vi "全局F参数.vi"() -> ()   [LabVIEW 2018]
panel:
  in  "选项卡控件":enum32{"1#", "2#", "3#"}(tab)
  in  "1#轮盘关开Pr":T1={"选择"=enum."Fx", "系数x"=1.0, "系数+"=1.0, "上限"=4.3, "下限"=3.7, "Ymax"=50.0, "Ymin"=-50.0, "点数"=1000.0, "锁系数x"=1.0, "锁上限"=0.4, "锁下限"=0.6, "锁系数+"=1.0, "起点"=0.20000000298023224, "终点"=0.6499999761581421, "锁起点"=0.05000000074505806, "锁终点"=0.20000000298023224, "上参考"=4.3, "下参考"=3.7, "基准"=3.7} {"系数+" format="%.3f"; "基准" format="%.2f"; "下参考" format="%.2f"; "上参考" format="%.2f"; "锁终点" format="%.2f"; "锁起点" format="%.2f"; "终点" format="%.2f"; "起点" format="%.2f"; "锁系数+" format="%.3f"; "锁下限" format="%.2f"; "锁上限" format="%.2f"; "锁系数x" format="%.3f"; "下限" format="%.2f"; "上限" format="%.2f"; "系数x" format="%.3f"}
  in  "1#轮盘开关Pr":T1={"选择"=enum."Fx", "系数x"=1.0, "系数+"=1.0, "上限"=4.3, "下限"=3.7, "Ymax"=50.0, "Ymin"=-50.0, "点数"=1000.0, "锁系数x"=1.0, "锁上限"=0.4, "锁下限"=0.6, "锁系数+"=1.0, "起点"=0.20000000298023224, "终点"=0.6499999761581421, "锁起点"=0.05000000074505806, "锁终点"=0.20000000298023224, "上参考"=4.3, "下参考"=3.7, "基准"=3.7} {"系数+" format="%.3f"; "基准" format="%.2f"; "下参考" format="%.2f"; "上参考" format="%.2f"; "锁终点" format="%.2f"; "锁起点" format="%.2f"; "终点" format="%.2f"; "起点" format="%.2f"; "锁系数+" format="%.3f"; "锁下限" format="%.2f"; "锁上限" format="%.2f"; "锁系数x" format="%.3f"; "下限" format="%.2f"; "上限" format="%.2f"; "系数x" format="%.3f"}
  in  "1#拨钮右左Pr":T1={"选择"=enum."Fx", "系数x"=1.0, "系数+"=1.0, "上限"=2.55, "下限"=2.05, "Ymax"=5.0, "Ymin"=-5.0, "点数"=1000.0, "锁系数x"=1.0, "锁上限"=0.4, "锁下限"=0.6, "锁系数+"=1.0, "起点"=0.0, "终点"=0.0, "锁起点"=0.05000000074505806, "锁终点"=0.20000000298023224, "上参考"=4.3, "下参考"=3.7, "基准"=3.7} {"系数+" format="%.3f"; "锁终点" format="%.2f"; "锁起点" format="%.2f"; "锁系数+" format="%.3f"; "锁下限" format="%.2f"; "锁上限" format="%.2f"; "锁系数x" format="%.3f"; "基准" format="%.2f"; "下参考" format="%.2f"; "上参考" format="%.2f"; "终点" format="%.2f"; "起点" format="%.2f"; "下限" format="%.2f"; "上限" format="%.2f"; "系数x" format="%.3f"}
  in  "1#拨钮左右Pr":T1={"选择"=enum."Fx", "系数x"=1.0, "系数+"=1.0, "上限"=2.55, "下限"=2.05, "Ymax"=5.0, "Ymin"=-5.0, "点数"=1000.0, "锁系数x"=1.0, "锁上限"=0.4, "锁下限"=0.6, "锁系数+"=1.0, "起点"=0.0, "终点"=0.0, "锁起点"=0.05000000074505806, "锁终点"=0.20000000298023224, "上参考"=4.3, "下参考"=3.7, "基准"=3.7} {"系数+" format="%.3f"; "锁终点" format="%.2f"; "锁起点" format="%.2f"; "锁系数+" format="%.3f"; "锁下限" format="%.2f"; "锁上限" format="%.2f"; "锁系数x" format="%.3f"; "基准" format="%.2f"; "下参考" format="%.2f"; "上参考" format="%.2f"; "终点" format="%.2f"; "起点" format="%.2f"; "下限" format="%.2f"; "上限" format="%.2f"; "系数x" format="%.3f"}
  in  "1#拨钮下上Pr":T1={"选择"=enum."Fx", "系数x"=1.0, "系数+"=1.0, "上限"=2.55, "下限"=2.05, "Ymax"=5.0, "Ymin"=-5.0, "点数"=1000.0, "锁系数x"=1.0, "锁上限"=0.4, "锁下限"=0.6, "锁系数+"=1.0, "起点"=0.0, "终点"=0.0, "锁起点"=0.05000000074505806, "锁终点"=0.20000000298023224, "上参考"=4.3, "下参考"=3.7, "基准"=3.7} {"系数+" format="%.3f"; "锁终点" format="%.2f"; "锁起点" format="%.2f"; "锁系数+" format="%.3f"; "锁下限" format="%.2f"; "锁上限" format="%.2f"; "锁系数x" format="%.3f"; "基准" format="%.2f"; "下参考" format="%.2f"; "上参考" format="%.2f"; "终点" format="%.2f"; "起点" format="%.2f"; "下限" format="%.2f"; "上限" format="%.2f"; "系数x" format="%.3f"}
  in  "1#拨钮上下Pr":T1={"选择"=enum."Fx", "系数x"=1.0, "系数+"=1.0, "上限"=2.55, "下限"=2.05, "Ymax"=5.0, "Ymin"=-5.0, "点数"=1000.0, "锁系数x"=1.0, "锁上限"=0.4, "锁下限"=0.6, "锁系数+"=1.0, "起点"=0.0, "终点"=0.0, "锁起点"=0.05000000074505806, "锁终点"=0.20000000298023224, "上参考"=4.3, "下参考"=3.7, "基准"=3.7} {"系数+" format="%.3f"; "锁终点" format="%.2f"; "锁起点" format="%.2f"; "锁系数+" format="%.3f"; "锁下限" format="%.2f"; "锁上限" format="%.2f"; "锁系数x" format="%.3f"; "基准" format="%.2f"; "下参考" format="%.2f"; "上参考" format="%.2f"; "终点" format="%.2f"; "起点" format="%.2f"; "下限" format="%.2f"; "上限" format="%.2f"; "系数x" format="%.3f"}
  in  "2#轮盘关开Pr":T1={"选择"=enum."Fx", "系数x"=1.0, "系数+"=1.0, "上限"=4.3, "下限"=3.7, "Ymax"=50.0, "Ymin"=-50.0, "点数"=1000.0, "锁系数x"=1.0, "锁上限"=0.4, "锁下限"=0.6, "锁系数+"=1.0, "起点"=0.20000000298023224, "终点"=0.6499999761581421, "锁起点"=0.05000000074505806, "锁终点"=0.20000000298023224, "上参考"=4.3, "下参考"=3.7, "基准"=3.7} {"系数+" format="%.3f"; "基准" format="%.2f"; "下参考" format="%.2f"; "上参考" format="%.2f"; "锁终点" format="%.2f"; "锁起点" format="%.2f"; "终点" format="%.2f"; "起点" format="%.2f"; "锁系数+" format="%.3f"; "锁下限" format="%.2f"; "锁上限" format="%.2f"; "锁系数x" format="%.3f"; "下限" format="%.2f"; "上限" format="%.2f"; "系数x" format="%.3f"}
  in  "2#轮盘开关Pr":T1={"选择"=enum."Fx", "系数x"=1.0, "系数+"=1.0, "上限"=4.3, "下限"=3.7, "Ymax"=50.0, "Ymin"=-50.0, "点数"=1000.0, "锁系数x"=1.0, "锁上限"=0.4, "锁下限"=0.6, "锁系数+"=1.0, "起点"=0.20000000298023224, "终点"=0.6499999761581421, "锁起点"=0.05000000074505806, "锁终点"=0.20000000298023224, "上参考"=4.3, "下参考"=3.7, "基准"=3.7} {"系数+" format="%.3f"; "基准" format="%.2f"; "下参考" format="%.2f"; "上参考" format="%.2f"; "锁终点" format="%.2f"; "锁起点" format="%.2f"; "终点" format="%.2f"; "起点" format="%.2f"; "锁系数+" format="%.3f"; "锁下限" format="%.2f"; "锁上限" format="%.2f"; "锁系数x" format="%.3f"; "下限" format="%.2f"; "上限" format="%.2f"; "系数x" format="%.3f"}
  in  "2#拨钮右左Pr":T1={"选择"=enum."Fx", "系数x"=1.0, "系数+"=1.0, "上限"=2.55, "下限"=2.05, "Ymax"=5.0, "Ymin"=-5.0, "点数"=1000.0, "锁系数x"=1.0, "锁上限"=0.4, "锁下限"=0.6, "锁系数+"=1.0, "起点"=0.0, "终点"=0.0, "锁起点"=0.05000000074505806, "锁终点"=0.20000000298023224, "上参考"=4.3, "下参考"=3.7, "基准"=3.7} {"系数+" format="%.3f"; "锁终点" format="%.2f"; "锁起点" format="%.2f"; "锁系数+" format="%.3f"; "锁下限" format="%.2f"; "锁上限" format="%.2f"; "锁系数x" format="%.3f"; "基准" format="%.2f"; "下参考" format="%.2f"; "上参考" format="%.2f"; "终点" format="%.2f"; "起点" format="%.2f"; "下限" format="%.2f"; "上限" format="%.2f"; "系数x" format="%.3f"}
  in  "2#拨钮左右Pr":T1={"选择"=enum."Fx", "系数x"=1.0, "系数+"=1.0, "上限"=2.55, "下限"=2.05, "Ymax"=5.0, "Ymin"=-5.0, "点数"=1000.0, "锁系数x"=1.0, "锁上限"=0.4, "锁下限"=0.6, "锁系数+"=1.0, "起点"=0.0, "终点"=0.0, "锁起点"=0.05000000074505806, "锁终点"=0.20000000298023224, "上参考"=4.3, "下参考"=3.7, "基准"=3.7} {"系数+" format="%.3f"; "锁终点" format="%.2f"; "锁起点" format="%.2f"; "锁系数+" format="%.3f"; "锁下限" format="%.2f"; "锁上限" format="%.2f"; "锁系数x" format="%.3f"; "基准" format="%.2f"; "下参考" format="%.2f"; "上参考" format="%.2f"; "终点" format="%.2f"; "起点" format="%.2f"; "下限" format="%.2f"; "上限" format="%.2f"; "系数x" format="%.3f"}
  in  "2#拨钮下上Pr":T1={"选择"=enum."Fx", "系数x"=1.0, "系数+"=1.0, "上限"=2.55, "下限"=2.05, "Ymax"=5.0, "Ymin"=-5.0, "点数"=1000.0, "锁系数x"=1.0, "锁上限"=0.4, "锁下限"=0.6, "锁系数+"=1.0, "起点"=0.0, "终点"=0.0, "锁起点"=0.05000000074505806, "锁终点"=0.20000000298023224, "上参考"=4.3, "下参考"=3.7, "基准"=3.7} {"系数+" format="%.3f"; "锁终点" format="%.2f"; "锁起点" format="%.2f"; "锁系数+" format="%.3f"; "锁下限" format="%.2f"; "锁上限" format="%.2f"; "锁系数x" format="%.3f"; "基准" format="%.2f"; "下参考" format="%.2f"; "上参考" format="%.2f"; "终点" format="%.2f"; "起点" format="%.2f"; "下限" format="%.2f"; "上限" format="%.2f"; "系数x" format="%.3f"}
  in  "2#拨钮上下Pr":T1={"选择"=enum."Fx", "系数x"=1.0, "系数+"=1.0, "上限"=2.55, "下限"=2.05, "Ymax"=5.0, "Ymin"=-5.0, "点数"=1000.0, "锁系数x"=1.0, "锁上限"=0.4, "锁下限"=0.6, "锁系数+"=1.0, "起点"=0.0, "终点"=0.0, "锁起点"=0.05000000074505806, "锁终点"=0.20000000298023224, "上参考"=4.3, "下参考"=3.7, "基准"=3.7} {"系数+" format="%.3f"; "锁终点" format="%.2f"; "锁起点" format="%.2f"; "锁系数+" format="%.3f"; "锁下限" format="%.2f"; "锁上限" format="%.2f"; "锁系数x" format="%.3f"; "基准" format="%.2f"; "下参考" format="%.2f"; "上参考" format="%.2f"; "终点" format="%.2f"; "起点" format="%.2f"; "下限" format="%.2f"; "上限" format="%.2f"; "系数x" format="%.3f"}
  in  "3#轮盘关开Pr":T1={"选择"=enum."Fx", "系数x"=1.0, "系数+"=1.0, "上限"=4.3, "下限"=3.7, "Ymax"=50.0, "Ymin"=-50.0, "点数"=1000.0, "锁系数x"=1.0, "锁上限"=0.4, "锁下限"=0.6, "锁系数+"=1.0, "起点"=0.20000000298023224, "终点"=0.6499999761581421, "锁起点"=0.05000000074505806, "锁终点"=0.20000000298023224, "上参考"=4.3, "下参考"=3.7, "基准"=3.7} {"系数+" format="%.3f"; "基准" format="%.2f"; "下参考" format="%.2f"; "上参考" format="%.2f"; "锁终点" format="%.2f"; "锁起点" format="%.2f"; "终点" format="%.2f"; "起点" format="%.2f"; "锁系数+" format="%.3f"; "锁下限" format="%.2f"; "锁上限" format="%.2f"; "锁系数x" format="%.3f"; "下限" format="%.2f"; "上限" format="%.2f"; "系数x" format="%.3f"}
  in  "3#轮盘开关Pr":T1={"选择"=enum."Fx", "系数x"=1.0, "系数+"=1.0, "上限"=4.3, "下限"=3.7, "Ymax"=50.0, "Ymin"=-50.0, "点数"=1000.0, "锁系数x"=1.0, "锁上限"=0.4, "锁下限"=0.6, "锁系数+"=1.0, "起点"=0.20000000298023224, "终点"=0.6499999761581421, "锁起点"=0.05000000074505806, "锁终点"=0.20000000298023224, "上参考"=4.3, "下参考"=3.7, "基准"=3.7} {"系数+" format="%.3f"; "基准" format="%.2f"; "下参考" format="%.2f"; "上参考" format="%.2f"; "锁终点" format="%.2f"; "锁起点" format="%.2f"; "终点" format="%.2f"; "起点" format="%.2f"; "锁系数+" format="%.3f"; "锁下限" format="%.2f"; "锁上限" format="%.2f"; "锁系数x" format="%.3f"; "下限" format="%.2f"; "上限" format="%.2f"; "系数x" format="%.3f"}
  in  "3#拨钮右左Pr":T1={"选择"=enum."Fx", "系数x"=1.0, "系数+"=1.0, "上限"=2.55, "下限"=2.05, "Ymax"=5.0, "Ymin"=-5.0, "点数"=1000.0, "锁系数x"=1.0, "锁上限"=0.4, "锁下限"=0.6, "锁系数+"=1.0, "起点"=0.0, "终点"=0.0, "锁起点"=0.05000000074505806, "锁终点"=0.20000000298023224, "上参考"=4.3, "下参考"=3.7, "基准"=3.7} {"系数+" format="%.3f"; "锁终点" format="%.2f"; "锁起点" format="%.2f"; "锁系数+" format="%.3f"; "锁下限" format="%.2f"; "锁上限" format="%.2f"; "锁系数x" format="%.3f"; "基准" format="%.2f"; "下参考" format="%.2f"; "上参考" format="%.2f"; "终点" format="%.2f"; "起点" format="%.2f"; "下限" format="%.2f"; "上限" format="%.2f"; "系数x" format="%.3f"}
  in  "3#拨钮左右Pr":T1={"选择"=enum."Fx", "系数x"=1.0, "系数+"=1.0, "上限"=2.55, "下限"=2.05, "Ymax"=5.0, "Ymin"=-5.0, "点数"=1000.0, "锁系数x"=1.0, "锁上限"=0.4, "锁下限"=0.6, "锁系数+"=1.0, "起点"=0.0, "终点"=0.0, "锁起点"=0.05000000074505806, "锁终点"=0.20000000298023224, "上参考"=4.3, "下参考"=3.7, "基准"=3.7} {"系数+" format="%.3f"; "锁终点" format="%.2f"; "锁起点" format="%.2f"; "锁系数+" format="%.3f"; "锁下限" format="%.2f"; "锁上限" format="%.2f"; "锁系数x" format="%.3f"; "基准" format="%.2f"; "下参考" format="%.2f"; "上参考" format="%.2f"; "终点" format="%.2f"; "起点" format="%.2f"; "下限" format="%.2f"; "上限" format="%.2f"; "系数x" format="%.3f"}
  in  "3#拨钮下上Pr":T1={"选择"=enum."Fx", "系数x"=1.0, "系数+"=1.0, "上限"=2.55, "下限"=2.05, "Ymax"=5.0, "Ymin"=-5.0, "点数"=1000.0, "锁系数x"=1.0, "锁上限"=0.4, "锁下限"=0.6, "锁系数+"=1.0, "起点"=0.0, "终点"=0.0, "锁起点"=0.05000000074505806, "锁终点"=0.20000000298023224, "上参考"=4.3, "下参考"=3.7, "基准"=3.7} {"系数+" format="%.3f"; "锁终点" format="%.2f"; "锁起点" format="%.2f"; "锁系数+" format="%.3f"; "锁下限" format="%.2f"; "锁上限" format="%.2f"; "锁系数x" format="%.3f"; "基准" format="%.2f"; "下参考" format="%.2f"; "上参考" format="%.2f"; "终点" format="%.2f"; "起点" format="%.2f"; "下限" format="%.2f"; "上限" format="%.2f"; "系数x" format="%.3f"}
  in  "3#拨钮上下Pr":T1={"选择"=enum."Fx", "系数x"=1.0, "系数+"=1.0, "上限"=2.55, "下限"=2.05, "Ymax"=5.0, "Ymin"=-5.0, "点数"=1000.0, "锁系数x"=1.0, "锁上限"=0.4, "锁下限"=0.6, "锁系数+"=1.0, "起点"=0.0, "终点"=0.0, "锁起点"=0.05000000074505806, "锁终点"=0.20000000298023224, "上参考"=4.3, "下参考"=3.7, "基准"=3.7} {"系数+" format="%.3f"; "锁终点" format="%.2f"; "锁起点" format="%.2f"; "锁系数+" format="%.3f"; "锁下限" format="%.2f"; "锁上限" format="%.2f"; "锁系数x" format="%.3f"; "基准" format="%.2f"; "下参考" format="%.2f"; "上参考" format="%.2f"; "终点" format="%.2f"; "起点" format="%.2f"; "下限" format="%.2f"; "上限" format="%.2f"; "系数x" format="%.3f"}
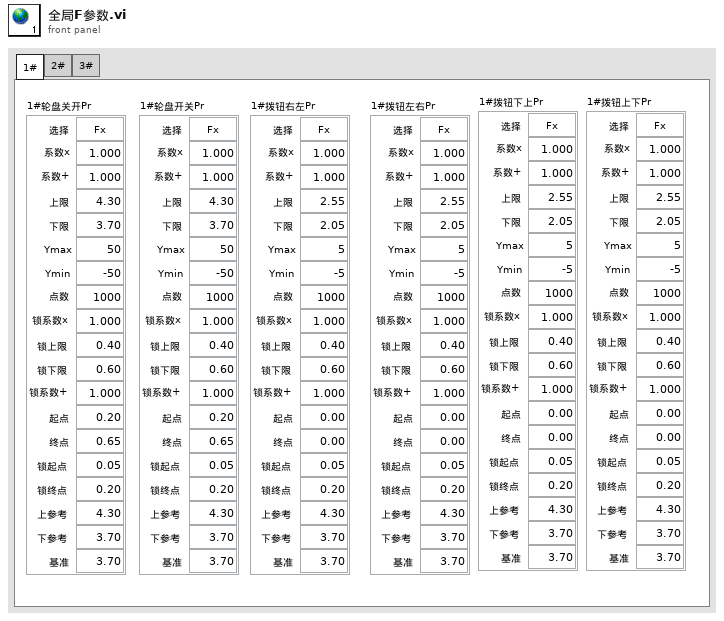
[diagram p1: front panel]
types:
  T1 = cluster{"选择":enum16{"Fx", "Fy", "Fz", "Mx", "My", "Mz"}, "系数x":sgl, "系数+":sgl, "上限":sgl, "下限":sgl, "Ymax":dbl, "Ymin":dbl, "点数":dbl, "锁系数x":sgl, "锁上限":sgl, "锁下限":sgl, "锁系数+":sgl, "起点":dbl, "终点":dbl, "锁起点":dbl, "锁终点":dbl, "上参考":sgl, "下参考":sgl, "基准":sgl}
diagram:
